vi "LJstreamM process data.vi"(6 "Disable Scaling":bool, 9 "Channel Config":T1={"# Channels"=4, "+Ch"=["0", "1", "2", "3", "4", "5", "6", "7"], "-Ch (U3)"=["31", "31", "31", "31", "31", "31", "31", "31"], "Ranges (UE9)"=[0, 0, 0, 0, 0, 0, 0, 0], "Scaling Equation"=["y=v0", "y=v1", "y=v2", "y=v3", "y=v4", "y=v5", "y=v6", "y=v7"]} {"Ranges (UE9)" items=["LJ_rgBIP5V", "LJ_rgUNI5V", "LJ_rgUNI2P5V", "LJ_rgUNI1P25V", "LJ_rgUNIP625V"]}, 11 "Voltages":dbl[][](array[numeric]) format="%.3f") -> (2 "Volts,Scaled Averages":dbl[][](array[numeric]) format="%.3f", 3 "Scaled Data":dbl[][](array[numeric]) format="%.3f")   [LabVIEW 2022 SP3]
uses:
  <vilib>/Analysis/baseanly.llb/Mean (DBL).vi
  <vilib>/Analysis/NI_AALBase.lvlib
panel:
  out "ms":u32
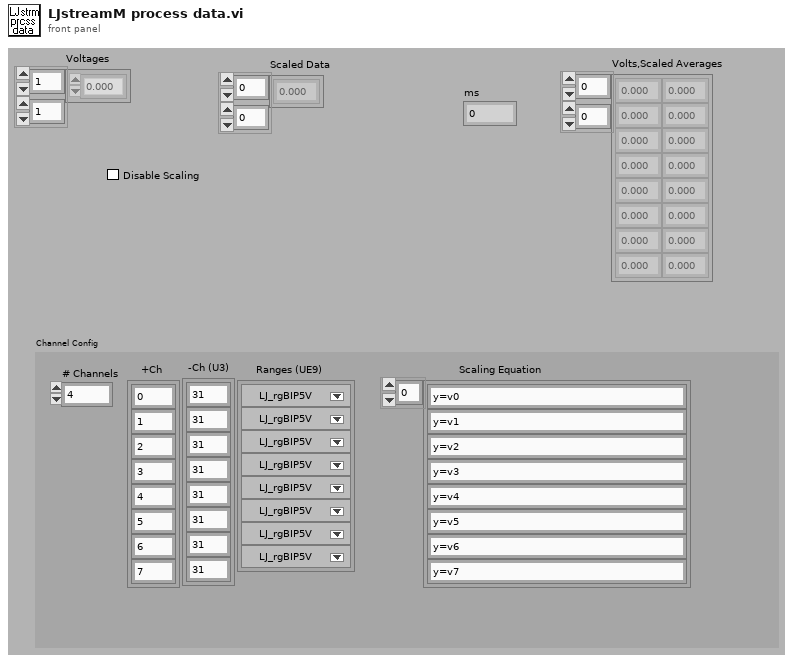
[diagram p1: front panel]
types:
  T1 = cluster{"# Channels":i32, "+Ch":string[], "-Ch (U3)":string[], "Ranges (UE9)":u16[], "Scaling Equation":string[]}
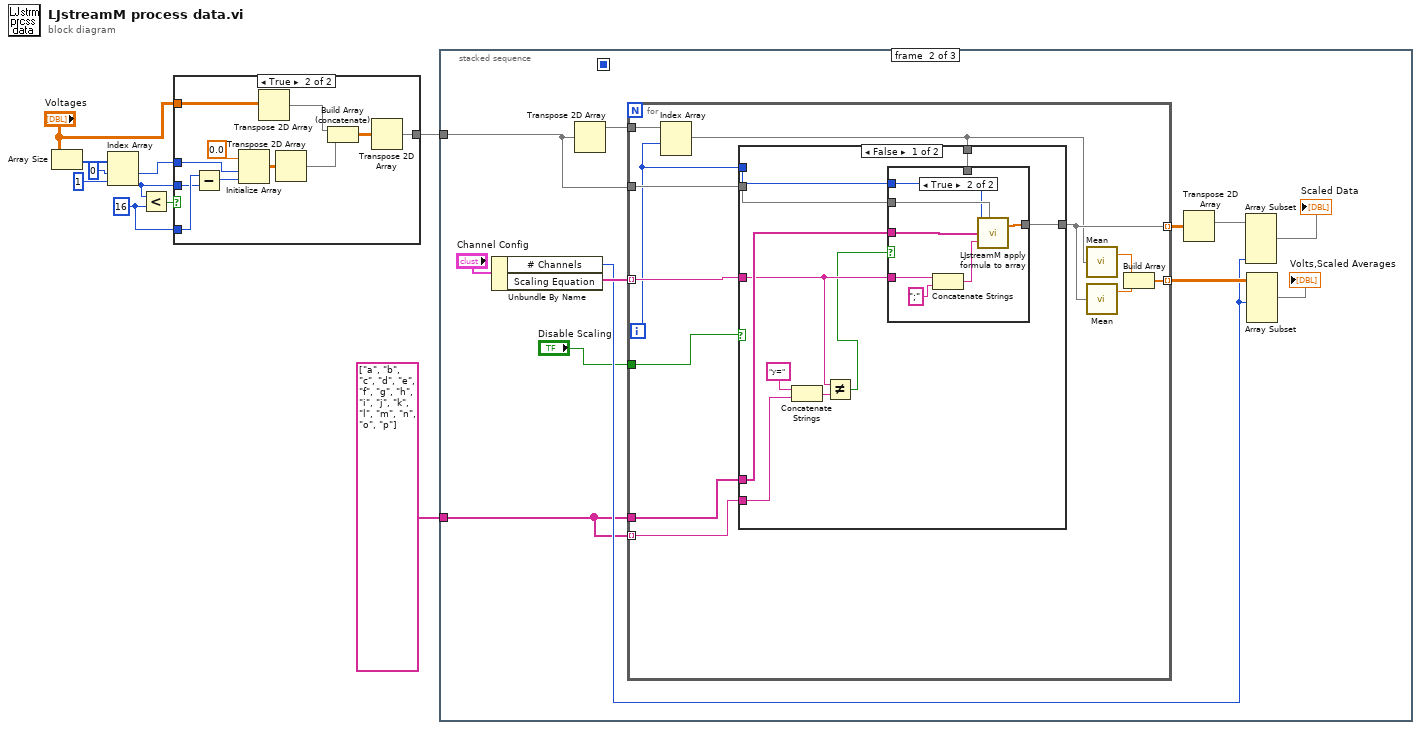
[diagram p0: block diagram]
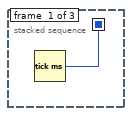
[diagram p3: hidden frame]
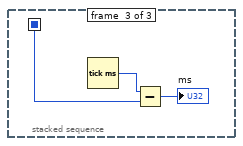
[diagram p6: hidden frame]
diagram:
  w6 = 16 ("y")
  n1 = Array Size(array="Voltages") -> (size(s)=w8:i32[])
  n2 = Index Array(array=w8, index #1=0 ("Index"), index #2=1 ("Index")) -> (element #1=w4:i32, element #2=w5:i32)
  n3 = Less?(x=w5, y=w6) -> (x < y?=w7:bool)
  n4 = case shown="True" w7 {
    tunnel: w6 -> [_ w22]
    tunnel: w5 -> [_ w21]
    tunnel: w4 -> [_ w20]
    tunnel: "Voltages" -> [w11 w17]
    tunnel: [w11 w14] -> w2
    frame False {
    }
    frame True {
      n5 = Subtract(x=w22, y=w21) -> (x-y=w19:i32)
      n6 = Initialize Array(0.0, w20, w19) -> (w13:dbl[][])
      n7 = Transpose 2D Array(2D array=w17) -> (transposed array=w16:dbl[][])
      n8 = Transpose 2D Array(2D array=w13) -> (transposed array=w12:dbl[][])
      n9 = Build Array (concatenate)(w16, w12) -> (w15:dbl[][])
      n10 = Transpose 2D Array(2D array=w15) -> (transposed array=w14:dbl[][])
    }
  }
  n11 = stacked-sequence {
    seq-local: [w23 _ _] -> [_ _ w68]
    tunnel: w2 -> [_ w31 _]
    tunnel: string[] ["a", "b", "c", "d", "e", "f", "g", "h", "i", "j", "k", "l", "m", "n", "o", "p"] ("Variables Input") -> [_ w25 _]
    frame #0 {
      n12 = Tick Count (ms)() -> (millisecond timer value=w23:u32)
    }
    frame #1 {
      n13 = Unbundle By Name("Channel Config") -> ("# Channels"=w26:i32, "Scaling Equation"=w32:string[])
      n14 = Transpose 2D Array(2D array=w31) -> (transposed array=w34:dbl[][])
      n15 = for {
        tunnel: w31 -> [w43]
        tunnel: w32 -> [w42] mode=indexing
        tunnel: [w44] -> w35 mode=indexing
        tunnel: [w45] -> w30 mode=indexing
        tunnel: w34 -> [w41]
        tunnel: w25 -> [w38]
        tunnel: w25 -> [w37] mode=indexing
        tunnel: "Disable Scaling" -> [w36]
        i -> [w39]
        n16 = Index Array(array=w41, index (row)=w39) -> (element=w40:dbl[])  [unwired: 1 in]
        n17 = case shown="False" w36 {
          tunnel: [w57 w66] -> w44
          tunnel: w43 -> [w56 _]
          tunnel: w42 -> [w51 _]
          tunnel: w40 -> [w48 w66]
          tunnel: w39 -> [w55 _]
          tunnel: w38 -> [w54 _]
          tunnel: w37 -> [w50 _]
          frame False {
            n18 = Concatenate Strings("y=", w50) -> (w52:string)
            n19 = Not Equal?(x=w51, y=w52) -> (x != y?=w49:bool)
            n20 = case shown="True" w49 {
              tunnel: [w58 w65] -> w57
              tunnel: w56 -> [_ w64]
              tunnel: w55 -> [_ w61]
              tunnel: w54 -> [_ w60]
              tunnel: w51 -> [_ w59]
              tunnel: w48 -> [w58 _]
              frame False {
              }
              frame True {
                n21 = Concatenate Strings(w59, ";" ("Substring")) -> (w63:string)
                n22 = call "LJstreamM apply formula to array.vi"("Index"=w61, "Input Values"=w64, "Variables Input"=w60, "formula"=w63) -> ("Output Values"=w65:dbl[])  [unwired: 1 in, 1 out]
              }
            }
          }
          frame True {
          }
        }
        n23 = call-poly <vilib>:"Mean.vi"("X"=w40) -> ("mean"=w47:dbl)  [unwired: 1 out]
        n24 = call-poly <vilib>:"Mean.vi"("X"=w44) -> ("mean"=w46:dbl)  [unwired: 1 out]
        n25 = Build Array(w47, w46) -> (w45:dbl[])
      }
      n26 = Transpose 2D Array(2D array=w35) -> (transposed array=w28:dbl[][])
      n27 = Array Subset(array=w28, length (col)=w26) -> (→"Scaled Data":dbl[][])  [unwired: 3 in]
      n28 = Array Subset(array=w30, length (row)=w26) -> (→"Volts,Scaled Averages":dbl[][])  [unwired: 3 in]
    }
    frame #2 {
      n29 = Tick Count (ms)() -> (millisecond timer value=w69:u32)
      n30 = Subtract(x=w69, y=w68) -> (x-y=→"ms":u32)
    }
  }
